vi "Shield.vi"   [LabVIEW 2013]
uses:
  State_Machine_Enum.ctl
  <vilib>/Rock Robotics/WPI/Solenoid/WPI_SolenoidValue.ctl
  RefnameEnum.ctl
  Robot Global Data.vi
  <vilib>/Rock Robotics/WPI/Solenoid/WPI_SolenoidSetEnum.vi
types:
  T1 = typedef "State_Machine_Enum.ctl" = enum16{"Idle", "Start", "Do", "Stop", "Init"}
  T2 = typedef "WPI_SolenoidValue.ctl" = enum16{"Off", "On", "Forward", "Reverse"}
  T3 = typedef "RefnameEnum.ctl" = enum16{"FireLauncher", "Climber", "Shield", "TankDrive", "DriveEncoderL", "DriveEncoderR", "LauncherMotorRPM", "LauncherEncoderAnalog", "LauncherEncoderRPM", "ShooterLS", "DriveAlignLSLeft", "DriveAlignLSRight", "ClimbingLS", "LauncherEncoderAngle", "LauncherMotorAngle", "Gamepad1", "Gamepad2", "Compressor", "ClimbWeightSol3", "ClimbWeightSol4"}
  T4 = typedef "WPI_SolenoidDevRef.ctl" = cluster{"DevStatus":errorcluster, "Solenoid Module":T5, "Forward Solenoid Channel":T6, "Reverse Solenoid Channel":T6}
  T5 = typedef "FPGA_TypedefSolenoidModule.ctl" = enum16{"Solenoid Module 1", "Solenoid Module 2"}
  T6 = typedef "WPI_SolenoidChannel.ctl" = enum8{"Solenoid 1", "Solenoid 2", "Solenoid 3", "Solenoid 4", "Solenoid 5", "Solenoid 6", "Solenoid 7", "Solenoid 8", "Invalid"}
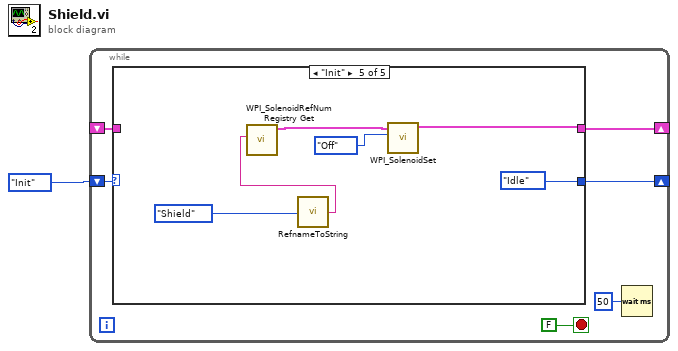
[diagram p0: block diagram]
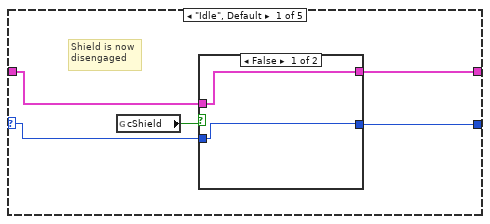
[diagram p2: hidden frame]
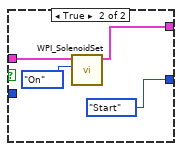
[diagram p3: hidden frame]
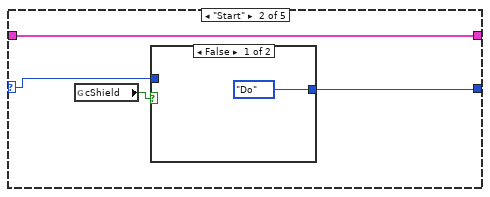
[diagram p4: hidden frame]
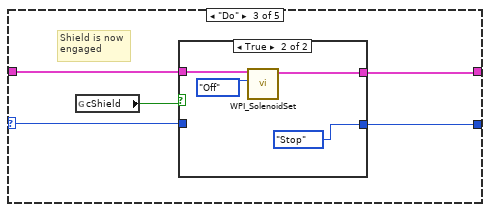
[diagram p6: hidden frame]
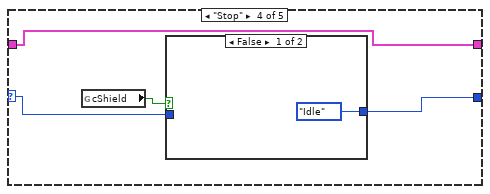
[diagram p8: hidden frame]
diagram:
  n1 = while {
    shift-right: [w6] -> _
    shift-left: State_Machine_Enum."Init" ("State") -> [w7]
    shift-right: [w5] -> _
    shift-left: _ -> [w4]
    stop <- FALSE stop-if-true
    n2 = case shown="\"Init\"" w7 {
      selector: w7 -> [w8 w19 w25 w37 _]
      tunnel: [w9 w20 w26 w38 State_Machine_Enum."Idle" ("State")] -> w6
      tunnel: [w10 w22 w27 w36 w45] -> w5
      tunnel: w4 -> [w11 w22 w28 w36 _]
      frame "Idle", Default {
        # "Shield is now\ndisengaged"
        n3 = global read "Robot Global Data.vi" "cShield"() -> (w12:bool)
        n4 = case shown="False" w12 {
          tunnel: w11 -> [w13 w18]
          tunnel: [w13 w17] -> w10
          tunnel: [w14 State_Machine_Enum."Start" ("State")] -> w9
          tunnel: w8 -> [w14 _]
          frame False {
          }
          frame True {
            n5 = call-poly <vilib>:"WPI_SolenoidSet.vi"("Value"=WPI_SolenoidValue."On", "SolenoidDevRef"=w18) -> ("SolenoidDevRef"=w17:T4)  [unwired: 8 in, 1 out]
          }
        }
      }
      frame "Start" {
        n6 = global read "Robot Global Data.vi" "cShield"() -> (w21:bool)
        n7 = case shown="False" w21 {
          tunnel: [State_Machine_Enum."Do" ("State") w24] -> w20
          tunnel: w19 -> [_ w24]
          frame False {
          }
          frame True {
          }
        }
      }
      frame "Do" {
        # "Shield is now\nengaged"
        n8 = global read "Robot Global Data.vi" "cShield"() -> (w29:bool)
        n9 = case shown="True" w29 {
          tunnel: w28 -> [w31 w35]
          tunnel: [w31 w34] -> w27
          tunnel: [w30 State_Machine_Enum."Stop" ("State")] -> w26
          tunnel: w25 -> [w30 _]
          frame False {
          }
          frame True {
            n10 = call-poly <vilib>:"WPI_SolenoidSet.vi"("Value"=WPI_SolenoidValue."Off", "SolenoidDevRef"=w35) -> ("SolenoidDevRef"=w34:T4)  [unwired: 8 in, 1 out]
          }
        }
      }
      frame "Stop" {
        n11 = global read "Robot Global Data.vi" "cShield"() -> (w39:bool)
        n12 = case shown="False" w39 {
          tunnel: [State_Machine_Enum."Idle" ("State") w41] -> w38
          tunnel: w37 -> [_ w41]
          frame False {
          }
          frame True {
          }
        }
      }
      frame "Init" {
        n13 = call "RefnameToString.vi"("Enum"=RefnameEnum."Shield") -> ("Refname"=w42:string)
        n14 = call <vilib>:"WPI_SolenoidRefNum Registry Get.vi"("refnum name"=w42) -> ("SolenoidDevRef"=w46:T4)  [unwired: 9 in, 1 out]
        n15 = call-poly <vilib>:"WPI_SolenoidSet.vi"("Value"=WPI_SolenoidValue."Off", "SolenoidDevRef"=w46) -> ("SolenoidDevRef"=w45:T4)  [unwired: 8 in, 1 out]
      }
    }
    n16 = Wait (ms)(milliseconds to wait=u32 50) -> ()  [unwired: 1 out]
  }
